vi "refresh trigger out before integration.vi"(8 "error in (no error)":errorcluster, 11 "LineCCD in":refnum<class "LineCCD.lvclass">) -> (0 "error out":errorcluster, 3 "LineCCD out":refnum<class "LineCCD.lvclass">)   [LabVIEW 2012, in "LineCCD.lvclass"]
uses:
  LineCCD.lvclass
  LineCCD.lvclass/LineCCD.ctl
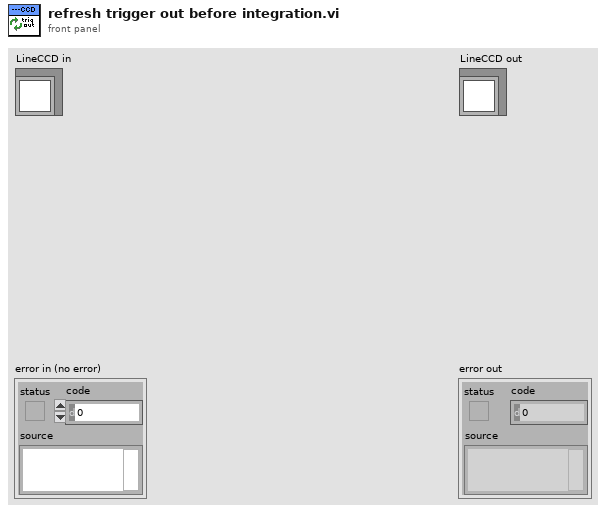
[diagram p1: front panel]
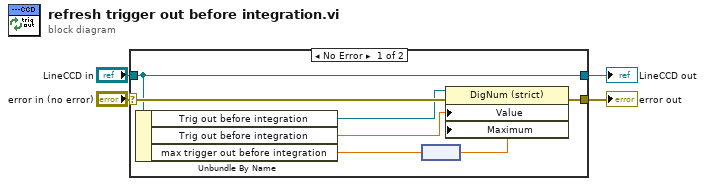
[diagram p0: block diagram]
diagram:
  n1 = case shown="No Error" "error in (no error)" {
    selector: "error in (no error)" -> [w11 w13]
    tunnel: [w10 w13] -> w3
    tunnel: [w9 w12] -> w1
    tunnel: "LineCCD in" -> [w9 w12]
    frame No Error {
      n2 = Unbundle By Name(w9) -> ("Trig out before integration"=w8:refnum<vi>, "Trig out before integration"=w7:dbl[unit], "max trigger out before integration"=w6:dbl[unit])
      n3 = node(w6) -> (w5:dbl)
      n4 = property class="DigNum (strict)"(reference=w8, error in=w11, "Value"=w7, "Maximum"=w5) -> (error out=w10:errorcluster)  [unwired: 1 out]
    }
    frame Error {
    }
  }
  "error out" <- w3
  "LineCCD out" <- w1
